vi "Dashboard Main.vi"() -> ()   [LabVIEW 2016]
uses:
  <vilib>/Rock Robotics/WPI/Camera/WPI_CameraExposure Values.ctl
  <vilib>/Rock Robotics/WPI/Camera/WPI_CameraWhite Balance Values.ctl
  <vilib>/Utility/miscctls.llb/LVRowAndColumnTypeDef.ctl
  <vilib>/event_ctls.llb/eventvkey.ctl
  <vilib>/Rock Robotics/Network Tables/NT Read Numeric Array.vi
  <vilib>/Rock Robotics/WPI/Dashboard/WPI_DashboardLogging Global.vi
  <vilib>/Rock Robotics/Network Tables/NT Read Boolean.vi
panel:
  in  "Camera Settings Right":T1={"Frame Rate"=15, "Compression"=30, "Size"=1, "DB Camera Config"=FALSE} {"Frame Rate" scale=1.0..30.0; "Compression" scale=100.0..-1.0; "Size" items=["640x480", "320x240", "160x120"]}
  in  "Camera Name Right":string(combo)="No Camera Selection"
  out "Camera Info":cluster{"Mbps LED":bool, "Mbps":dbl, "fps":dbl} {"fps" format="%#.1g"; "Mbps" format="%#.1g"}
  in  "Camera Settings":T1={"Frame Rate"=10, "Compression"=30, "Size"=1, "DB Camera Config"=FALSE} {"Frame Rate" scale=1.0..30.0; "Compression" scale=100.0..-1.0; "Size" items=["640x480", "320x240", "160x120"]}
  in  "TCP":refnum<k5>
  in  "Rec Mode":enum32{"Stop", "Record", "Playback"}(radio)
  out "Robot IP":string="0.0.0.0"
  out "Image Message":string="Timeout in Camera Communications"
  in  "Dashboard Tab":T2(tab)
  in  "Take Picture":bool
  in  "Vision Target":enum16{"Pegs", "Boiler", "Gears"}(ring)
  in  "Select Auto":string(combo)="Select Autonomous ..."
  out "NT Connection":bool
  out "MotorChart R":cluster{"Numeric":dbl, "Numeric":dbl}(graph)
  out "MotorChart L":cluster{"Numeric":dbl, "Numeric":dbl}(graph)
  out "MotorSliders R":cluster{"MotorSlide1":dbl, "MotorSlide2":dbl} {"MotorSlide2" scale=-1.0..1.0 scale format="%#_2e"; "MotorSlide1" scale=-1.0..1.0 scale format="%#_2e"}
  out "MotorSliders L":cluster{"MotorSlide1":dbl, "MotorSlide2":dbl} {"MotorSlide2" scale=-1.0..1.0 scale format="%#_2e"; "MotorSlide1" scale=-1.0..1.0 scale format="%#_2e"}
  out "Gyro":dbl(knob) scale=0.0..360.0
  out "JS1 Z":dbl(slide) scale=-1.0..1.0 scale format="%#_2e"
  out "JS1 Graph":cluster{"X":dbl, "Y":dbl}[](graph)
  out "JS1 Buttons":T3
  out "JS2 Z":dbl(slide) scale=-1.0..1.0 scale format="%#_2e"
  out "JS2 Graph":cluster{"X":dbl, "Y":dbl}[](graph)
  out "JS2 Buttons":T3
  out "Mode":T4(ring)=enum."Disconnected"
  in  "gear/peg":bool
  out "Binary Image":T5(plugin-control)
  out "Camera Image Right":T5(plugin-control)
  in  "DB/String 9":string
  in  "DB/String 8":string
  in  "DB/String 7":string
  in  "DB/String 6":string
  in  "DB/String 5":string
  in  "DB/String 4":string
  in  "DB/String 3":string
  in  "DB/String 2":string
  in  "DB/String 1":string
  in  "DB/String 0":string
  in  "DB/Slider 0":dbl(slide) scale=0.0..5.0
  in  "DB/Slider 1":dbl(slide) scale=0.0..5.0
  in  "DB/Slider 2":dbl(slide) scale=0.0..5.0
  in  "DB/Slider 3":dbl(slide) scale=0.0..5.0
  out "DB/LED 3":bool
  out "DB/LED 2":bool
  out "DB/LED 1":bool
  out "DB/LED 0":bool
  in  "DB/Button 3":bool
  in  "DB/Button 2":bool
  in  "DB/Button 1":bool
  in  "DB/Button 0":bool caption="New Name"
  in  "Test Slider":dbl(slide) scale=0.0..100.0 scale format="%#_3g"
  in  "On/Off":bool caption="Solenoid"
  in  "Test Name":u16(ring) items=["Select the test to run..."]
  in  "Test Tree":string(tree)
  in  "Motor":cluster{"Value":dbl, "Enable":bool} {"Value" scale=-1.0..1.0 scale format="%#_3g"}
  out "Progress":T6 {"Test Progress" scale=0.0..100.0}
  in  "Rev/Fwd":cluster{"Forward":bool, "Reverse":bool}
  in  "Test Ring":u16(ring) items=["Monochrome", "Color"]
  out "Cmd Status":string
  in  "Execute Command":bool
  in  "Command Params":string[][](table)
  in  "Command Selection":i32(listbox)
  in  "CheckList":i32(listbox)
  out "Tree":string(tree)
  out "Camera Image":T5(plugin-control)
  out "Background":bool
  in  "Camera Name":string(combo)="No Camera Selection"
  # "HW"
  # "HW"
  # "Joysticks"
  # "Drive Motors"
  # "Front"
  # "Right"
  # "Left"
  # "Back"
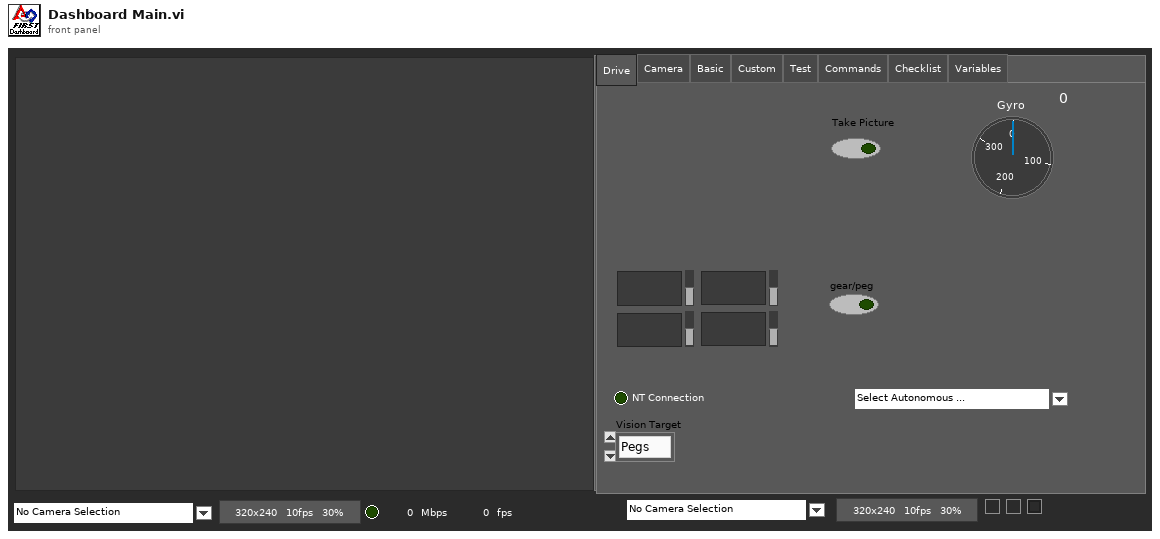
[diagram p1: front panel]
types:
  T1 = cluster{"Frame Rate":i32, "Compression":i32, "Size":u16, "DB Camera Config":bool}
  T2 = enum32{"Drive", "Camera", "Basic", "Custom", "Test", "Commands", "Checklist", "Variables"}
  T3 = cluster{bool, bool, bool, bool, bool, bool, bool, bool, bool, bool, bool, bool}
  T4 = enum8{"Tele-Op Disabled", "Tele-Op Enabled", "Auto Disabled", "Auto Enabled", "Test Disabled", "Test Enabled", "Disconnected", "No Code", "E-Stop"}
  T5 = typedef "IMAQ Image.ctl" = refnum<image>
  T6 = cluster{"Test Progress":u8, "Test Progress Text":string}
  T7 = typedef "Particle Parameters" = i32
  T8 = cluster{"IDs":cluster{"RPC field ID":u16, "Unique ID":u16}, "String":string}
  T9 = enum32{"Drive", "Basic", "Custom", "Test", "Checklist", "Variables"}
  T10 = typedef "Image Type" = u32
  T11 = cluster{"Error Strings":string, "Disable Counts":cluster{u16, u16}, "Rail Faults":cluster{u16, u16, u16}, "Robot IP":string, "DB Mode":u8, "Event Info":cluster{"Name":string, "Type":u8, "Number":u16, "Replay":u8}}
  T12 = cluster{"Storage":cluster{"Disk Free":u64, "RAM Block":u32, "RAM free":u32}, "CPU Utilization":cluster{"CPU % ISR":sgl, "CPU % Time Crit":sgl, "CPU % Timed Str":sgl, "CPU % High":sgl, "CPU % Above":sgl, "CPU % Normal":sgl, "CPU % Low":sgl}, "CAN":cluster{"% Bus Utilization":sgl, "Bus Off Cnt":u32, "TX_FIFO Full Cnt":u32, "Receive Error Cnt":u8, "Transmit Error Cnt":u8}, "HID":cluster{"HID Outputs":u32, "Rumble Low":u16, "Rumble High":u16}[]}
  T13 = cluster{"Status bits":cluster{"Test Mode":bool, "Autonomous":bool, "Enabled":bool, "Code Start":bool, "Brownout":bool, "Reserved 2":bool, "Reserved 3":bool, "E-Stop":bool}, "Code Trace":cluster{"Disabled":bool, "TeleOp":bool, "Auto":bool, "Test":bool}, "Controller Type":enum16{"unknown", "cRIO", "roboRio"}, "Code?":enum16{"unknown", "noCode", "code"}, "Battery V":dbl}
  T14 = cluster{"Control Bits":cluster{"TestMode":bool, "Autonomous":bool, "Enabled":bool, "FMS Present":bool, bool, bool, bool, "E-Stop":bool}, "Team Station ":u8, "Countdown":sgl, "Joystick Values":cluster{"Axes":dbl[], "Buttons":bool[], "POVs":i16[]}[]}
  T15 = cluster{"Axes":dbl[], "Buttons":bool[], "POVs":i16[]}[]
  T16 = cluster{"Axes":dbl[], "Buttons":bool[], "POVs":i16[]}
  T17 = cluster{"Buttons[0]":bool, "Buttons[1]":bool, "Buttons[2]":bool, "Buttons[3]":bool, "Buttons[4]":bool, "Buttons[5]":bool, "Buttons[6]":bool, "Buttons[7]":bool, "Buttons[8]":bool, "Buttons[9]":bool, "Buttons[10]":bool, "Buttons[11]":bool}
  T18 = cluster{"Camera Image":refnum<vi>, "Dashboard Tab":refnum<vi>, "Background":refnum<vi>, "Rec Mode":refnum<vi>, "Test Slider":refnum<vi>, "On/Off ":refnum<vi>, "Test Ring":refnum<vi>, "Rev/Fwd":refnum<vi>, "Test Name":refnum<vi>, "Motor":refnum<vi>, "Progress":refnum<vi>, "CheckList":refnum<vi>, "Tree":refnum<vi>, "Test Tree":refnum<vi>, "Command Params":refnum<vi>, "Command Selection":refnum<vi>, "Execute Command":refnum<vi>, "Cmd Status":refnum<vi>, "Camera Settings":refnum<vi>, "Camera Name":refnum<vi>, "Camera Info":refnum<vi>, "Camera Settings Right":refnum<vi>, "Camera Name Right":refnum<vi>, "Camera Image Right":refnum<vi>}
  T19 = typedef "WPI_CameraExposure Values.ctl" = enum16{"Auto", "Flicker-free 50 Hz", "Flicker-free 60 Hz", "Hold current", "Custom"}
  T20 = typedef "WPI_CameraWhite Balance Values.ctl" = enum16{"Auto", "Fixed indoor", "Fixed outdoor 1", "Fixed outdoor 2", "Fixed fluorescent 1", "Fixed fluorescent 2", "Hold current", "Custom"}
  T21 = cluster{"Exposure":T19, "Exposure (%)":dbl, "Brightness":i32, "White Balance":T20, "Color Temp (K)":dbl}
  T22 = cluster{"Left":dbl, "Top":dbl, "Right":dbl, "Bottom":dbl}
  T23 = cluster{"Numeric":dbl, "Numeric":dbl, "Numeric":dbl, "Numeric":dbl}
  T24 = cluster{"Operation":enum16{"Update", "Clear"}, "Color Box":u32}[]
  T25 = typedef "eventvkey.ctl" = enum16{"ASCII", "Enter", "Return", "Shift", "Ctrl", "Alt", "Cmd", "Opt", "Caps", "NumLock", "Clear", "Break", "Up", "Down", "Left", "Right", "Insert", "Delete", "Home", "End", "PageUp", "PageDown", "Escape", "Help", "Pause", "ScrollLock", "F1", "F2", "F3", "F4", "F5", "F6", "F7", "F8", "F9", "F10", "F11", "F12", "F13", "F14", "F15", "F16", "F17", "F18", "F19", "F20", "F21", "F22", "F23", "F24", "Play", "VolumeUp", "VolumeDown", "Mute", "Two Byte Char"}
  T26 = cluster{"Image Size":bool, "Image Type":bool, "Pixel Value":bool, "ROI Information":bool, "Zoom Factor":bool}
  T27 = cluster{"Operation":enum16{"Update", "Clear"}, "Color Box":u32}
  T28 = typedef "LVRowAndColumnTypeDef.ctl" = cluster{"Row":i32, "Column":i32}
  T29 = cluster{"Shift":bool, "Ctrl":bool, "Alt":bool, "Cmd":bool, "Opt":bool}
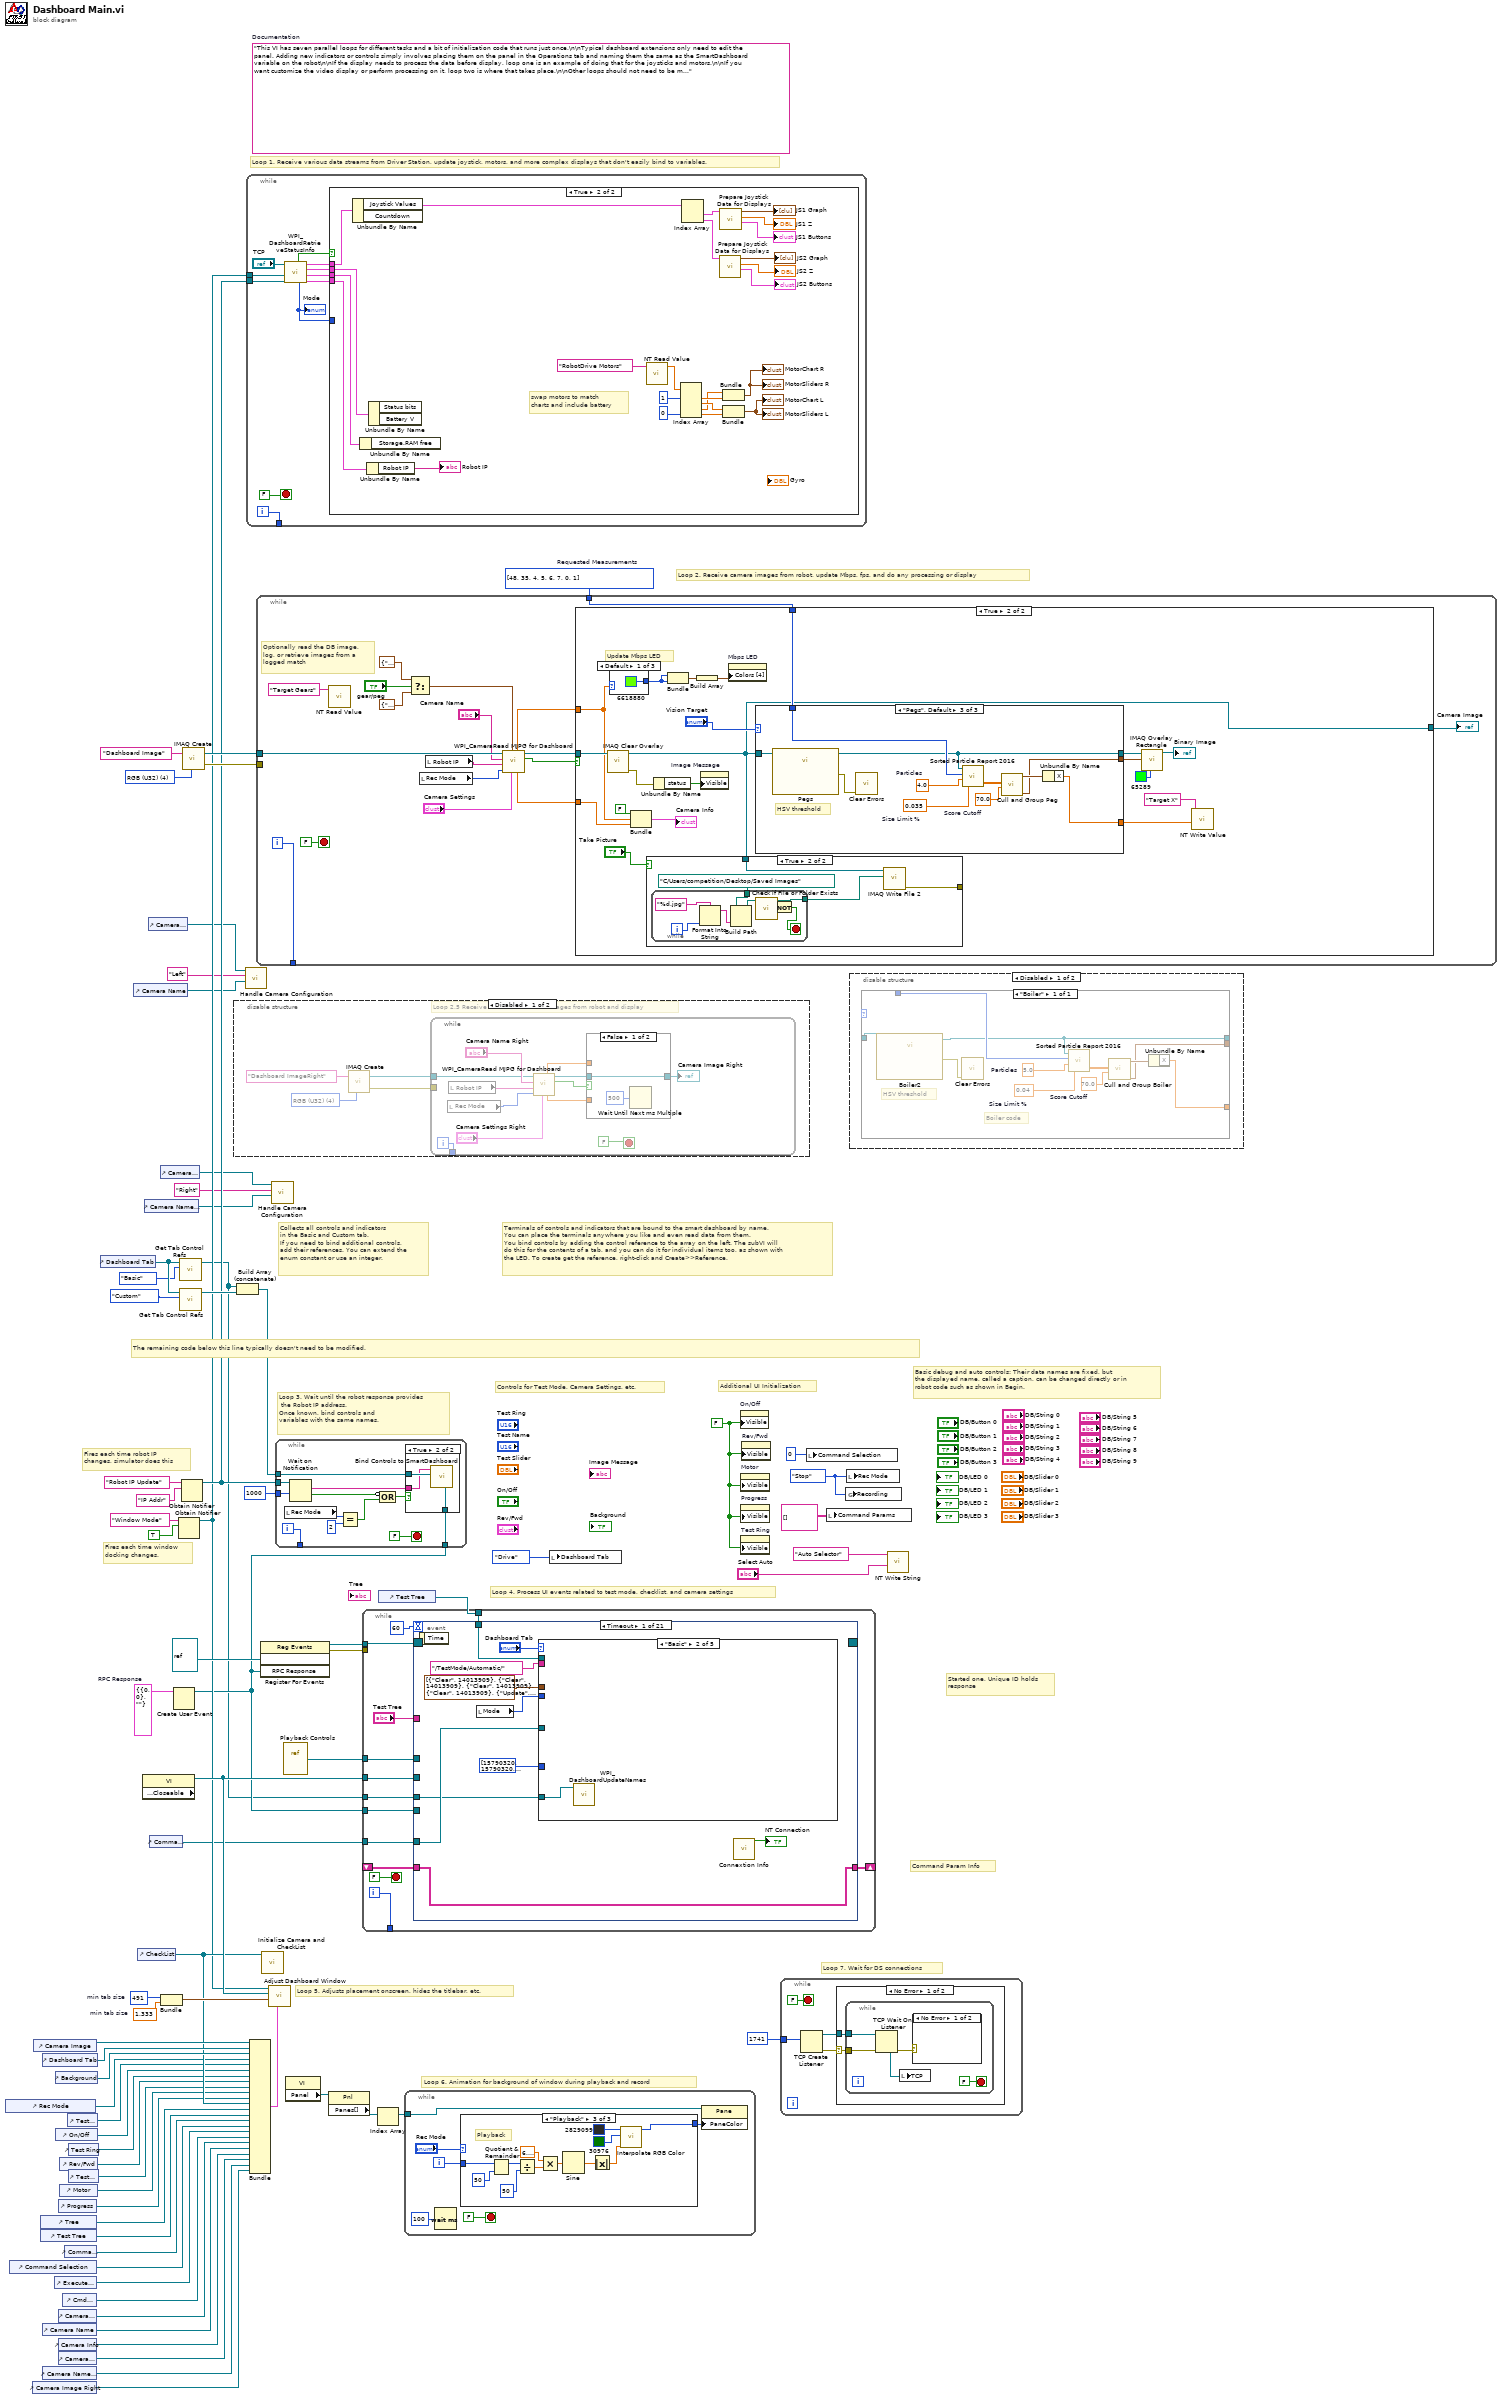
[diagram p0: block diagram]
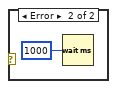
[diagram p5: hidden frame]
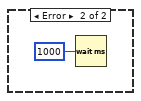
[diagram p6: hidden frame]
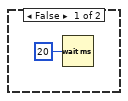
[diagram p7: hidden frame]
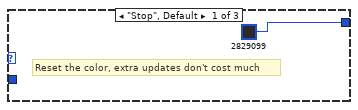
[diagram p8: hidden frame]
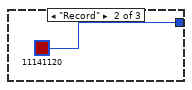
[diagram p9: hidden frame]
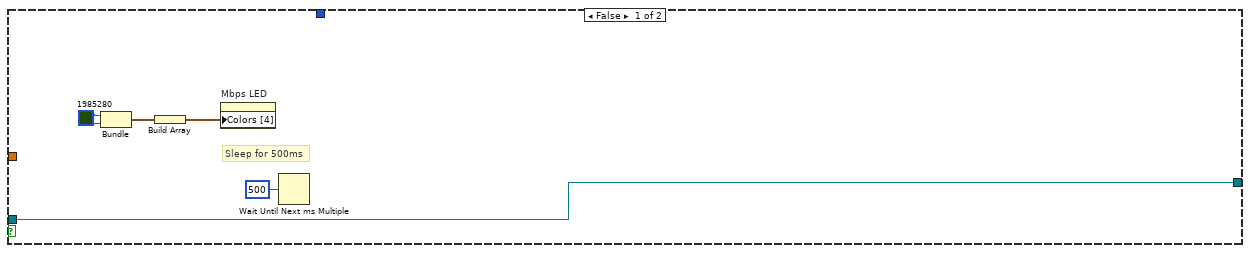
[diagram p11: hidden frame]
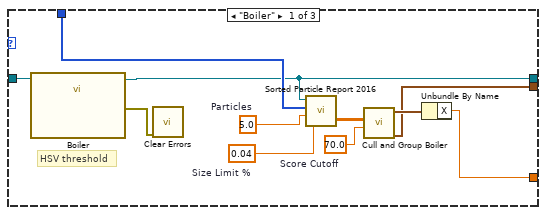
[diagram p13: hidden frame]
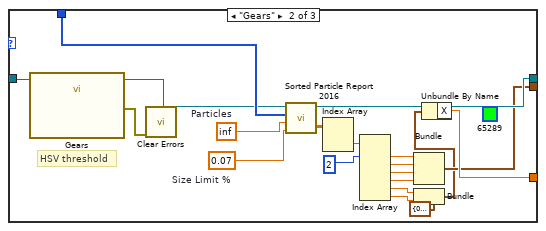
[diagram p14: hidden frame]
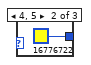
[diagram p15: hidden frame]
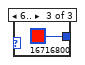
[diagram p16: hidden frame]
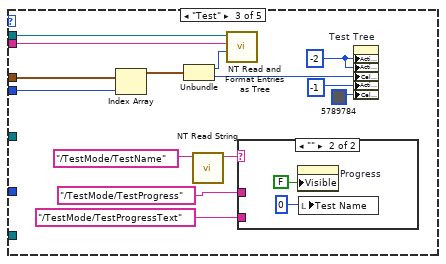
[diagram p18: hidden frame]
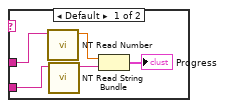
[diagram p19: hidden frame]
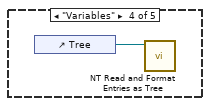
[diagram p20: hidden frame]
diagram:
  w1 = T7[] [48, 35, 4, 5, 6, 7, 0, 1] items=["Center of Mass X", "Center of Mass Y", "First Pixel X", "First Pixel Y", "Bounding Rect Left", "Bounding Rect Top", "Bounding Rect Right", "Bounding Rect Bottom", "Max Feret Diameter Start X", "Max Feret Diameter Start Y", "Max Feret Diameter End X", "Max Feret Diameter End Y", "Max Horiz. Segment Length Left", "Max Horiz. Segment Length Right", "Max Horiz. Segment Length Row", "-", "Bounding Rect Width", "Bounding Rect Height", "Bounding Rect Diagonal", "Perimeter", "Convex Hull Perimeter", "Holes' Perimeter", "Max Feret Diameter", "Equivalent Ellipse Major Axis", "Equivalent Ellipse Minor Axis", "Equivalent Ellipse Minor Axis (Feret)", "Equivalent Rect Long Side", "Equivalent Rect Short Side", "Equivalent Rect Diagonal", "Equivalent Rect Short Side (Feret)", "Average Horiz. Segment Length", "Average Vert. Segment Length", "Hydraulic Radius", "Waddel Disk Diameter", "-", "Area", "Holes' Area", "Particle & Holes' Area", "Convex Hull Area", "Image Area", "-", "Number of Holes", "Number of Horiz. Segments", "Number of Vert. Segments", "-", "Orientation", "Max Feret Diameter Orientation", "-", "% Area/Image Area", "% Area/(Particle & Holes' Area)", "Ratio of Equivalent Ellipse Axes", "Ratio of Equivalent Rect Sides", "-", "Elongation Factor", "Compactness Factor", "Heywood Circularity Factor", "Type Factor", "-", "Sum X", "Sum Y", "Sum XX", "Sum XY", "Sum YY", "Sum XXX", "Sum XXY", "Sum XYY", "Sum YYY", "-", "Moment of Inertia XX", "Moment of Inertia XY", "Moment of Inertia YY", "Moment of Inertia XXX", "Moment of Inertia XXY", "Moment of Inertia XYY", "Moment of Inertia YYY", "Norm. Moment of Inertia XX", "Norm. Moment of Inertia XY", "Norm. Moment of Inertia YY", "Norm. Moment of Inertia XXX", "Norm. Moment of Inertia XXY", "Norm. Moment of Inertia XYY", "Norm. Moment of Inertia YYY", "Hu Moment 1", "Hu Moment 2", "Hu Moment 3", "Hu Moment 4", "Hu Moment 5", "Hu Moment 6", "Hu Moment 7"]  # Requested Measurements
  w23 = T8 {"IDs"={"RPC field ID"=0, "Unique ID"=0}, "String"=""}  # RPC Response
  w48 = 491  # min tab size
  w47 = 1.333  # min tab size
  w55 = enum32{"Stop", "Record", "Playback"}."Stop" ("Rec Mode")
  w30 = FALSE ("Visible")
  (unwired) "This VI has seven parallel loops for different tasks and a bit of initialization code that runs just once.\n\nTypical dashboard extensions only need to edit the panel. Adding new indicators or controls simply involves placing them on the panel in the Operations tab and naming them the same as the SmartDashboard variable on the robot\n\nIf the display needs to process the data before display, loop one is an example of doing that for the joysticks and motors.\n\nIf you want customize the video display or perform processing on it, loop two is where that takes place.\n\nOther loops should not need to be modified. They are pretty standard, and document the task they perform."  # Documentation
  w72 = T10 4 items=["Grayscale (U8)", "Grayscale (I16)", "Grayscale (SGL)", "Complex (CSG)", "RGB (U32)", "HSL (U32)", "RGB (U64)"] ("Image Type")
  # "Command Param Info"
  # "Started one, Unique ID holds\nresponse"
  # "Loop 7. Wait for DS connections"
  # "Basic debug and auto controls: Their data names are fixed, but\nthe displayed name, called a caption, can be changed directly or in\nrobot code such as shown in Begin."
  # "Controls for Test Mode, Camera Settings, etc."
  # "Additional UI Initialization"
  # "Loop 6. Animation for background of window during playback and record"
  # "Fires each time robot IP\nchanges, simulator does this"
  # "Fires each time window\ndocking changes."
  # "Collects all controls and indicators\nin the Basic and Custom tab.\nIf you need to bind additional controls,\nadd their references. You can extend the\nenum constant or use an integer."
  # "The remaining code below this line typically doesn't need to be modified."
  # "Loop 4. Process UI events related to test mode, checklist, and camera settings"
  # "Terminals of controls and indicators that are bound to the smart dashboard by name.\nYou can place the terminals anywhere you like and even read data from them.\nYou bind controls by adding the control reference to the array on the left. The subVI will\ndo this for the contents of a tab, and you can do it for individual items too, as shown with\nthe LED. To create get the reference, right-click and Create>>Reference."
  # "Loop 3. Wait until the robot response provides\n the Robot IP address.\nOnce known, bind controls and\nvariables with the same names."
  # "Loop 5. Adjusts placement onscreen, hides the titlebar, etc."
  # "Loop 1. Receive various data streams from Driver Station, update joystick, motors, and more complex displays that don't easily bind to variables."
  # "Loop 2. Receive camera images from robot, update Mbps, fps, and do any processing or display"
  n1 = control-ref of="Rec Mode"() -> (w36:refnum<vi>)
  n2 = control-ref of="Command Selection"() -> (w22:refnum<vi>)
  n3 = control-ref of="Camera Image Right"() -> (w2:refnum<vi>)
  n4 = control-ref of="Camera Image"() -> (w50:refnum<vi>)
  n5 = control-ref of="Tree"() -> (w40:refnum<vi>)
  n6 = control-ref of="Test Tree"() -> (w39:refnum<vi>)
  n7 = control-ref of="Dashboard Tab"() -> (w49:refnum<vi>)
  n8 = control-ref of="Camera Name"() -> (w13:refnum<vi>)
  n9 = control-ref of="Camera Name Right"() -> (w3:refnum<vi>)
  n10 = control-ref of="Execute Command"() -> (w24:refnum<vi>)
  n11 = control-ref of="Background"() -> (w45:refnum<vi>)
  n12 = control-ref of="On/Off"() -> (w34:refnum<vi>)
  n13 = control-ref of="Progress"() -> (w31:refnum<vi>)
  n14 = control-ref of="Camera Settings"() -> (w14:refnum<vi>)
  n15 = control-ref of="Camera Info"() -> (w12:refnum<vi>)
  n16 = control-ref of="Camera Settings Right"() -> (w4:refnum<vi>)
  n17 = control-ref of="Rev/Fwd"() -> (w32:refnum<vi>)
  n18 = control-ref of="Motor"() -> (w37:refnum<vi>)
  n19 = control-ref of="Cmd Status"() -> (w18:refnum<vi>)
  n20 = control-ref of="Command Params"() -> (w25:refnum<vi>)
  n21 = control-ref of="Test Slider"() -> (w35:refnum<vi>)
  n22 = control-ref of="Test Ring"() -> (w33:refnum<vi>)
  n23 = control-ref of="Test Name"() -> (w38:refnum<vi>)
  n24 = control-ref of="Dashboard Tab"() -> (w53:refnum<vi>)
  n25 = control-ref of="Camera Name"() -> (w15:refnum<vi>)
  n26 = control-ref of="CheckList"() -> (w41:refnum<vi>)
  n27 = property class="VI" props=["Front Panel.Closeable"]() -> (reference out=w54:refnum<vi>)  [unwired: 2 in, 2 out]
  n28 = control-ref of="Camera Name Right"() -> (w7:refnum<vi>)
  n29 = control-ref of="Camera Settings"() -> (w16:refnum<vi>)
  n30 = control-ref of="Command Params"() -> (w17:refnum<vi>)
  n31 = control-ref of="Camera Settings Right"() -> (w8:refnum<vi>)
  n32 = Bundle("min tab size"=w48, "min tab size"=w47) -> (w46:cluster{"min tab size":i32, "min tab size":dbl})  [unwired: 1 in]
  n33 = Create User Event(user event datatype=w23) -> (user event=w19:refnum<user-event>)  [unwired: 1 in, 1 out]
  n34 = Obtain Notifier(name (unnamed)="Window Mode", notification data type=TRUE) -> (notifier out=w28:refnum<notifier>)  [unwired: 2 in, 2 out]
  n35 = call <vilib>:"Get Tab Control Refs.vi"("Page Index"=T9."Basic" ("Dashboard Tab"), "TabControl in"=w53) -> ("ControlsOnPage"=w11:refnum<vi>[])  [unwired: 9 in]
  n36 = call <vilib>:"Get Tab Control Refs.vi"("Page Index"=T9."Custom" ("Dashboard Tab"), "TabControl in"=w53) -> ("ControlsOnPage"=w52:refnum<vi>[])  [unwired: 9 in]
  n37 = Obtain Notifier(name (unnamed)="Robot IP Update", notification data type="IP Addr" ("name (unnamed)")) -> (notifier out=w29:refnum<notifier>)  [unwired: 2 in, 2 out]
  n38 = call "IMAQ Create"("Image Name"="Dashboard Image", "Image Type"=w72) -> ("New Image"=w70:T5, "error out"=w69:errorcluster)  [unwired: 2 in, 1 out]
  n39 = disable-structure shown="Disabled" {
    frame Disabled {
      w75 = T10 4 items=["Grayscale (U8)", "Grayscale (I16)", "Grayscale (SGL)", "Complex (CSG)", "RGB (U32)", "HSL (U32)", "RGB (U64)"] ("Image Type")
      # "Loop 2.5 Receive additional camera images from robot and display"
      n40 = call "IMAQ Create"("Image Name"="Dashboard ImageRight", "Image Type"=w75) -> ("New Image"=w74:T5, "error out"=w73:errorcluster)  [unwired: 2 in, 1 out]
      n41 = while {
        tunnel: w74 -> [w87]
        tunnel: w73 -> [_]
        tunnel: [w81] -> _
        i -> [w81]
        stop <- FALSE stop-if-true
        n42 = local read "Rec Mode"() -> (w85:enum32{"Stop", "Record", "Playback"})
        n43 = local read "Robot IP"() -> (w86:string)
        n44 = call <vilib>:"WPI_CameraRead MJPG for Dashboard.vi"("Camera Settings"="Camera Settings Right", "Rec Mode"=w85, "Robot IP"=w86, "Camera Name"="Camera Name Right", "Refnum in"=w87) -> ("Active"=w80:bool, "Refnum out"=w83:T5, "FPS"=w78:dbl, "Bandwidth (Mbps)"=w79:dbl)  [unwired: 3 in]
        n45 = case shown="False" w80 {
          tunnel: w83 -> [w89 w91]
          tunnel: w79 -> [_ _]
          tunnel: w78 -> [_ _]
          tunnel: [w89 w91] -> w77
          frame False {
            n46 = Wait Until Next ms Multiple(millisecond multiple=u32 500) -> ()  [unwired: 1 out]
          }
          frame True {
          }
        }
        "Camera Image Right" <- w77
      }
    }
    frame Enabled {
    }
  }
  n47 = Build Array (concatenate)(w11, w52) -> (w51:refnum<vi>[])
  n48 = call "Handle Camera Configuration.vi"("CameraNameRef"=w15, "Camera File Name"="Left", "ClusterRef"=w16) -> ()  [unwired: 9 in]
  n49 = while {
    tunnel: [w101] -> _
    tunnel: w29 -> [w95]
    tunnel: w28 -> [w92]
    i -> [w101]
    stop <- FALSE stop-if-true
    n50 = call <vilib>:"WPI_DashboardRetrieveStatusInfo.vi"("Binding Refnum"=w95, "Window Mode Notifier"=w92, "TCP Cnx"="TCP") -> ("Power and Errors"=w96:T11, "Robot Metrics"=w99:T12, "Status Info"=w100:T13, "Control Info"=w97:T14, "Robot Mode"=w94:T4, "Process?"=w98:bool)  [unwired: 3 in]
    "Mode" <- w94
    n51 = case shown="True" w98 {
      tunnel: w100 -> [_ w127]
      tunnel: w99 -> [_ w126]
      tunnel: w97 -> [_ w125]
      tunnel: w96 -> [_ w124]
      tunnel: w94 -> [_ _]
      frame False {
        n52 = Wait (ms)(milliseconds to wait=u32 20) -> ()  [unwired: 1 out]
      }
      frame True {
        # "swap motors to match\ncharts and include battery"
        n53 = Unbundle By Name(w125) -> ("Joystick Values"=w115:T15)  [unwired: 1 out]
        n54 = Unbundle By Name(w126) -> ()  [unwired: 1 out]
        n55 = Unbundle By Name(w124) -> ("Robot IP"=→"Robot IP":string)
        n56 = Unbundle By Name(w127) -> ()  [unwired: 2 out]
        n57 = call-poly <vilib>:"NT Read Value.vi"("Name"="RobotDrive Motors") -> ("Numeric Array"=w105:dbl[])  [unwired: 9 in, 1 out]
        n58 = Index Array(array=w105, index #1=1, index #4=0) -> (element #1=w119:dbl, element #2=w120:dbl, element #3=w118:dbl, element #4=w123:dbl)  [unwired: 2 in]
        n59 = Index Array(array=w115) -> (element #1=w114:T16, element #2=w110:T16)  [unwired: 2 in]
        n60 = call "Prepare Joystick Data for Displays.vi"("Joystick Values"=w110) -> ("Buttons"=→"JS2 Buttons":T17, "Z Axis"=→"JS2 Z":dbl, "Cartesian Data"=→"JS2 Graph":cluster{"X axis":dbl, "X axis":dbl}[])  [unwired: 8 in]
        n61 = call "Prepare Joystick Data for Displays.vi"("Joystick Values"=w114) -> ("Buttons"=→"JS1 Buttons":T17, "Z Axis"=→"JS1 Z":dbl, "Cartesian Data"=→"JS1 Graph":cluster{"X axis":dbl, "X axis":dbl}[])  [unwired: 8 in]
        n62 = Bundle("Numeric"=w118, "Numeric"=w119) -> (→"MotorChart R" →"MotorSliders R":cluster{"Numeric":dbl, "Numeric":dbl})  [unwired: 1 in]
        n63 = Bundle("Numeric"=w120, "Numeric"=w123) -> (→"MotorChart L" →"MotorSliders L":cluster{"Numeric":dbl, "Numeric":dbl})  [unwired: 1 in]
      }
    }
  }
  n64 = Bundle("Camera Image"=w50, "Dashboard Tab"=w49, "Background"=w45, "Rec Mode"=w36, "Test Slider"=w35, "On/Off"=w34, "Test Ring"=w33, "Rev/Fwd"=w32, "Test Name"=w38, "Motor"=w37, "Progress"=w31, "CheckList"=w41, "Tree"=w40, "Test Tree"=w39, "Command Params"=w25, "Command Selection"=w22, "Execute Command"=w24, "Cmd Status"=w18, "Camera Settings"=w14, "Camera Name"=w13, "Camera Info"=w12, "Camera Settings Right"=w4, "Camera Name Right"=w3, "Camera Image Right"=w2) -> (w42:T18)  [unwired: 1 in]
  n65 = while {
    tunnel: w70 -> [w143]
    tunnel: w69 -> [_]
    tunnel: [w144] -> _
    tunnel: w1 -> [w134]
    i -> [w144]
    stop <- FALSE stop-if-true
    # "Optionally read the DB image,\nlog, or retrieve images from a\nlogged match"
    n66 = call-poly <vilib>:"NT Read Value.vi"("Name"="Target Gears") -> ()  [unwired: 9 in, 2 out]
    n67 = Select(t=T21 {"Exposure"=enum."Custom", "Exposure (%)"=35.0, "Brightness"=50, "White Balance"=enum."Custom", "Color Temp (K)"=0.0} ("Bright"), s="gear/peg", f=T21 {"Exposure"=enum."Custom", "Exposure (%)"=0.0, "Brightness"=0, "White Balance"=enum."Custom", "Color Temp (K)"=0.0} ("Dark")) -> (s? t:f=w132:T21)
    n68 = local read "Rec Mode"() -> (w140:enum32{"Stop", "Record", "Playback"})
    n69 = local read "Robot IP"() -> (w139:string)
    n70 = call <vilib>:"WPI_CameraRead MJPG for Dashboard.vi"("Camera Settings"="Camera Settings", "Camera Settings 2"=w132, "Rec Mode"=w140, "Robot IP"=w139, "Camera Name"="Camera Name", "Refnum in"=w143) -> ("Active"=w142:bool, "Refnum out"=w129:T5, "FPS"=w141:dbl, "Bandwidth (Mbps)"=w138:dbl)  [unwired: 2 in]
    n71 = case shown="True" w142 {
      tunnel: w129 -> [w146 w166]
      tunnel: w138 -> [_ w163]
      tunnel: w141 -> [_ w164]
      tunnel: [w146 w153] -> w135
      tunnel: w134 -> [_ w160]
      frame False {
        w148 = u32 1985280 ("Color Box")
        # "Sleep for 500ms"
        n72 = Bundle("Color Box"=w148, "Color Box"=w148) -> (w149:cluster{"Color Box":u32, "Color Box":u32})  [unwired: 1 out]
        n73 = Build Array(w149) -> (w147:cluster{"Color Box":u32, "Color Box":u32}[])
        n74 = property on="Mbps LED" class="Bool (strict)"("Colors [4]"=w147) -> ()  [unwired: 2 in, 2 out]
        n75 = Wait Until Next ms Multiple(millisecond multiple=u32 500) -> ()  [unwired: 1 out]
      }
      frame True {
        # "Update Mbps LED"
        n76 = call "IMAQ Clear Overlay"("Image"=w166) -> ("error out"=w169:errorcluster, "Image Out"=w153:T5)  [unwired: 2 in, 7 out]
        n77 = case shown="Default" w163 {
          tunnel: [u32 6618880 ("Color Box") u32 16776722 ("Color Box") u32 16716800 ("Color Box")] -> w167
          frame Default {
          }
          frame 4, 5 {
          }
          frame 6.. {
          }
        }
        n78 = Bundle(FALSE, "Bandwidth (Mbps)"=w163, "FPS"=w164) -> (→"Camera Info":cluster{bool, "Bandwidth (Mbps)":dbl, "FPS":dbl})  [unwired: 1 in]
        n79 = case shown="True" "Take Picture" {
          tunnel: w153 -> [_ w174]
          tunnel: [_ w173] -> _
          frame False {
          }
          frame True {
            n80 = while {
              tunnel: path "C:/Users/competition/Desktop/Saved Images" ("base path") -> [w179]
              tunnel: [w177] -> w171
              i -> [w181]
              stop <- w176 stop-if-true
              n81 = Format Into String(format string="%d.jpg", w181) -> (resulting string=w180:string)  [unwired: 2 in, 1 out]
              n82 = Build Path(base path=w179, name or relative path=w180) -> (appended path=w178:path)
              n83 = call <vilib>:"Check if File or Folder Exists.vi"("path"=w178) -> ("file or folder exists?"=w182:bool, "dup path"=w177:path)  [unwired: 8 in, 1 out]
              n84 = Not(x=w182) -> (.not. x?=w176:bool)
            }
            n85 = call-poly "IMAQ Write File 2"("File Path"=w171, "Image"=w174) -> ("error out"=w173:errorcluster)  [unwired: 3 in, 6 out]
          }
        }
        n86 = Unbundle By Name(w169) -> ("status"=w170:bool)
        n87 = Bundle("Color Box"=w167, "Color Box"=w167) -> (w168:cluster{"Color Box":u32, "Color Box":u32})  [unwired: 1 out]
        n88 = Build Array(w168) -> (w165:cluster{"Color Box":u32, "Color Box":u32}[])
        n89 = property on="Image Message" class="Str"("Visible"=w170) -> ()  [unwired: 2 in, 2 out]
        n90 = property on="Mbps LED" class="Bool (strict)"("Colors [4]"=w165) -> ()  [unwired: 2 in, 2 out]
        n91 = case shown="\"Pegs\", Default" "Vision Target" {
          tunnel: w160 -> [w190 w207 w221]
          tunnel: [w186 w212 w220] -> w151
          tunnel: w153 -> [w185 w210 w219]
          tunnel: [w183 w206 w214] -> w156
          tunnel: [w184 w198 w215] -> w154
          frame "Boiler" {
            w188 = 70.0  # Score Cutoff
            w192 = 5.0  # Particles
            w191 = 0.04  # Size Limit %
            # "HSV threshold"
            n92 = call "Boiler"("Image In"=w185) -> ("Image Out"=w183:T5, "error out"=w193:errorcluster)  [unwired: 25 in]
            n93 = call <vilib>:"Clear Errors.vi"("error in (no error)"=w193) -> ()  [unwired: 5 in, 2 out]
            n94 = call "Sorted Particle Report 2016.vi"("Min Area Size %"=w191, "Particle Count Limit"=w192, "Pixel Measurements"=w190, "Image in"=w183) -> ("Sorted Data"=w189:dbl[][])  [unwired: 1 out]
            n95 = call "Cull and Group Boiler.vi"("Score Cutoff"=w188, "Sorted Data"=w189) -> ("Rect"=w184:T22, "Center"=w187:cluster{"X":dbl, "Y":dbl})  [unwired: 6 in, 2 out]
            n96 = Unbundle By Name(w187) -> ("X"=w186:dbl)
          }
          frame "Gears" {
            w209 = inf  # Particles
            w208 = 0.07  # Size Limit %
            (unwired) u32 65289 ("Color")
            # "HSV threshold"
            n97 = call "Gears"("Image In"=w210) -> ("Image Out"=w206:T5, "error out"=w211:errorcluster)  [unwired: 25 in]
            n98 = call <vilib>:"Clear Errors.vi"("error in (no error)"=w211) -> ()  [unwired: 5 in, 2 out]
            n99 = call "Sorted Particle Report 2016.vi"("Min Area Size %"=w208, "Particle Count Limit"=w209, "Pixel Measurements"=w207, "Image in"=w206) -> ("Sorted Data"=w205:dbl[][])  [unwired: 1 out]
            n100 = Index Array(array=w205) -> (element=w204:dbl[])  [unwired: 2 in]
            n101 = Index Array(array=w204, index #1=2 ("index")) -> (element #1=w202:dbl, element #2=w201:dbl, element #3=w200:dbl, element #4=w199:dbl, element #5=w196:dbl, element #6=w197:dbl)  [unwired: 5 in]
            n102 = Bundle("Numeric"=w202, "Numeric"=w201, "Numeric"=w200, "Numeric"=w199) -> (w198:T23)  [unwired: 1 in]
            n103 = Bundle(cluster=cluster{"X":dbl, "Y":dbl} {"X"=0.0, "Y"=0.0} ("input cluster"), "X"=w196, "Y"=w197) -> (w194:cluster{"X":dbl, "Y":dbl})
            n104 = Unbundle By Name(w194) -> ("X"=w212:dbl)
          }
          frame "Pegs", Default {
            w216 = 70.0  # Score Cutoff
            w223 = 4.0  # Particles
            w222 = 0.035  # Size Limit %
            # "HSV threshold"
            n105 = call "Pegs"("Image In"=w219) -> ("Image Out"=w214:T5, "error out"=w213:errorcluster)  [unwired: 25 in]
            n106 = call <vilib>:"Clear Errors.vi"("error in (no error)"=w213) -> ()  [unwired: 5 in, 2 out]
            n107 = call "Sorted Particle Report 2016.vi"("Min Area Size %"=w222, "Particle Count Limit"=w223, "Pixel Measurements"=w221, "Image in"=w214) -> ("Sorted Data"=w218:dbl[][])  [unwired: 1 out]
            n108 = call "Cull and Group Peg.vi"("Score Cutoff"=w216, "Sorted Data"=w218) -> ("Rect"=w215:T22, "Center"=w217:cluster{"X":dbl, "Y":dbl})  [unwired: 6 in, 2 out]
            n109 = Unbundle By Name(w217) -> ("X"=w220:dbl)
          }
        }
        n110 = call "IMAQ Overlay Rectangle"("Color"=u32 65289, "Rectangle"=w154, "Image"=w156) -> ("Image Out"=→"Binary Image":T5)  [unwired: 7 in, 1 out]
        n111 = call-poly <vilib>:"NT Write Value.vi"("Numeric"=w151, "Name"="Target X") -> ()  [unwired: 9 in, 1 out]
      }
    }
    "Camera Image" <- w135
  }
  n112 = register-events(refnum<vi> refnum, w19) -> (reference out=w59:refnum<event-registration>, error out=w58:errorcluster)  [unwired: 2 in]
  n113 = call "Initialize Camera and CheckList.vi"("ListBox in"=w41) -> ()  [unwired: 11 in]
  n114 = call "Adjust Dashboard Window.vi"("Sizing Refnums"=w42, "Size Constraints"=w46, "VI"=w54, "WIn Mode"=w28) -> ()  [unwired: 8 in]
  n115 = call "Handle Camera Configuration.vi"("CameraNameRef"=w7, "Camera File Name"="Right", "ClusterRef"=w8) -> ()  [unwired: 9 in]
  n116 = while {
    tunnel: w51 -> [w238]
    tunnel: w29 -> [w236]
    tunnel: [w234] -> _
    tunnel: u32 1000 ("milliseconds to wait") -> [w233]
    tunnel: w19 -> [w227]
    i -> [w234]
    stop <- FALSE stop-if-true
    n117 = local read "Rec Mode"() -> (w229:enum32{"Stop", "Record", "Playback"})
    n118 = Wait on Notification(notifier=w236, timeout in ms (-1)=w233) -> (notification=w235:string, timed out?=w231:bool)  [unwired: 2 in, 2 out]
    n119 = Equal?(x=w229, y=u16 2 ("Rec Mode")) -> (x = y?=w230:bool)
    n120 = Compound Arithmetic op=OR(invert w231, w230) -> (w232:bool)
    n121 = case shown="True" w232 {
      tunnel: w238 -> [_ w241]
      tunnel: w235 -> [_ w240]
      tunnel: w227 -> [_ w239]
      frame False {
      }
      frame True {
        n122 = call <vilib>:"Bind Controls to SmartDashboard.vi"("RPC ref"=w239, "Bound Control Refs"=w241, "Server IP Address"=w240) -> ()  [unwired: 9 in]
      }
    }
  }
  n123 = vi-ref "Playback Controls.vi"() -> (w60:refnum<vi>)
  n124 = property class="VI"() -> ("Panel"=w62:refnum<vi>)  [unwired: 2 in, 2 out]
  n125 = property class="Pnl"(reference=w62) -> ("Panes[]"=w63:refnum<vi>[])  [unwired: 1 in, 2 out]
  n126 = Index Array(array=w63) -> (element=w61:refnum<vi>)  [unwired: 1 in]
  n127 = control-ref of="Test Tree"() -> (w64:refnum<vi>)
  n128 = while {
    tunnel: [w251] -> _
    tunnel: w64 -> [w250]
    tunnel: w60 -> [w249]
    tunnel: w59 -> [w248]
    tunnel: w58 -> [_]
    tunnel: w54 -> [w247]
    tunnel: w19 -> [w246]
    tunnel: w17 -> [w245]
    shift-right: [w244] -> _
    shift-left: _ -> [w243]
    tunnel: w11 -> [w242]
    i -> [w251]
    stop <- FALSE stop-if-true
    n129 = event shown="[0] Timeout" {
      selector: w248 -> [_ _ _ _ _ _ _ _ _ _ _ _ _ _ _ _ _ _ _ _ _]
      dyn-events: [_ _ _ _ _ _ _ _ _ _ _ _ _ _ _ _ w507 _ _ _ _] -> _
      timeout: u32 60 ("milliseconds to wait") -> [_ _ _ _ _ _ _ _ _ _ _ _ _ _ _ _ _ _ _ _ _]
      tunnel: w250 -> [w263 _ _ _ _ _ _ _ _ _ _ _ _ _ _ _ _ _ _ _ _]
      tunnel: "Test Tree" -> [_ _ _ _ _ _ _ _ _ _ _ w474 w482 w484 w488 w496 _ _ _ _ _]
      tunnel: w249 -> [_ _ _ _ _ _ _ _ _ _ _ _ _ _ _ _ w509 _ w527 _ _]
      tunnel: w247 -> [_ _ _ _ _ _ _ _ _ _ _ _ _ _ _ _ w505 _ _ _ _]
      tunnel: w246 -> [_ _ _ _ _ _ _ _ _ _ _ _ _ _ _ _ w501 _ _ _ _]
      tunnel: w245 -> [w258 _ _ _ _ _ w425 _ _ _ _ _ _ _ _ _ _ _ _ _ _]
      tunnel: [w257 w302 w404 w409 w418 w422 w423 w432 w442 w449 w461 w473 w480 w483 w487 w495 w500 w522 w524 w528 w539] -> w244
      tunnel: w243 -> [w257 w302 w404 w409 w418 w422 w423 _ _ w449 w461 w473 w480 w483 w487 w495 w500 w522 w524 w528 w539]
      tunnel: w242 -> [w255 _ _ _ _ _ _ _ _ _ _ _ _ _ _ _ _ _ _ _ _]
      event Timeout {
        n130 = event-data() -> ()  [unwired: 1 in, 1 out]
        n131 = local read "Mode"() -> (w260:T4)
        n132 = case shown="\"Basic\"" "Dashboard Tab" {
          tunnel: w263 -> [_ _ w279 _ _]
          tunnel: "/TestMode/Automatic/" ("Name Pattern") -> [_ _ w278 _ _]
          tunnel: T24 [{"Operation"=enum."Clear", "Color Box"=14013909}, {"Operation"=enum."Clear", "Color Box"=14013909}, {"Operation"=enum."Clear", "Color Box"=14013909}, {"Operation"=enum."Clear", "Color Box"=14013909}, {"Operation"=enum."Update", "Color Box"=14013909}, {"Operation"=enum."Update", "Color Box"=16777215}, {"Operation"=enum."Clear", "Color Box"=14013909}, {"Operation"=enum."Clear", "Color Box"=14013909}, {"Operation"=enum."Clear", "Color Box"=14013909}] -> [_ _ w271 _ w295]
          tunnel: w260 -> [_ _ w270 _ w294]
          tunnel: u32[] [15790320, 15790320, 15790320, 15790320, 16777215, 16777215, 15790320, 15790320, 15790320] -> [_ _ _ _ w300]
          tunnel: w258 -> [_ _ _ _ w288]
          tunnel: w255 -> [_ w265 _ _ _]
          frame "Custom", Default {
          }
          frame "Basic" {
            n133 = call <vilib>:"WPI_DashboardUpdateNames.vi"("Controls on Tab"=w265) -> ()  [unwired: 11 in]
          }
          frame "Test" {
            w277 = -2 ("Active Item:Row Number")
            n134 = Index Array(array=w271, index=w270) -> (element=w272:T27)
            n135 = Unbundle(w272) -> ("Operation"=w273:enum16{"Update", "Clear"}, "Color Box"=w274:u32)
            n136 = call <vilib>:"NT Read String.vi"("Name"="/TestMode/TestName") -> ("String"=w268:string)  [unwired: 9 in, 1 out]
            n137 = call <vilib>:"NT Read and Format Entries as Tree.vi"("Operation"=w273, "Name Pattern"=w278, "Tree Refnum"=w279) -> ()  [unwired: 7 in, 2 out]
            n138 = case shown="\"\"" w268 {
              tunnel: "/TestMode/TestProgress" ("Name") -> [w281 _]
              tunnel: "/TestMode/TestProgressText" ("Name") -> [w280 _]
              frame Default {
                n139 = call <vilib>:"NT Read Number.vi"("Name"=w281) -> ("Numeric"=w282:dbl)  [unwired: 9 in, 1 out]
                n140 = call <vilib>:"NT Read String.vi"("Name"=w280) -> ("String"=w283:string)  [unwired: 9 in, 1 out]
                n141 = Bundle("Numeric"=w282, "String"=w283) -> (→"Progress":cluster{"Numeric":dbl, "String":string})  [unwired: 1 in]
              }
              frame "" {
                n142 = property on="Progress" class="Clust (strict)"("Visible"=FALSE) -> ()  [unwired: 2 in, 2 out]
                n143 = local write "Test Name"(u16 0) -> ()
              }
            }
            n144 = property on="Test Tree" class="Tree (strict)"("Active Item Row Number"=w277, "ActiveColNum"=w277, "CellBG"=w274, "Active Item Row Number"=-1 ("Active Item:Row Number"), "CellBG"=u32 5789784 ("Color Box")) -> ()  [unwired: 2 in, 2 out]
          }
          frame "Variables" {
            n145 = control-ref of="Tree"() -> (w287:refnum<vi>)
            n146 = call <vilib>:"NT Read and Format Entries as Tree.vi"("Tree Refnum"=w287) -> ()  [unwired: 9 in, 2 out]
          }
          frame "Commands" {
            w296 = u32 5789784 ("Color Box")
            w297 = T28 {"Row"=-1, "Column"=-2} ("Active Cell:Active Cell")
            w299 = T28 {"Row"=-2, "Column"=-2} ("Active Cell:Active Cell")
            n147 = Index Array(array=w300, index=w294) -> (element=w298:u32)
            n148 = Index Array(array=w295, index=w294) -> (element=w293:T27)
            n149 = Unbundle(w293) -> ("Operation"=w292:enum16{"Update", "Clear"})  [unwired: 1 out]
            n150 = local read "Command Selection"() -> (w291:i32)
            n151 = property on="Command Selection" class="MCListbox (strict)"("ActiveCell"=w299, "CellBG"=w298, "ActiveCell"=w297, "CellBG"=w296) -> ()  [unwired: 2 in, 2 out]
            n152 = call <vilib>:"WPI_DashboardUpdate RPC Info.vi"("Operation"=w292) -> ("update"=w290:bool, "commands"=w289:string[][])  [unwired: 9 in]
            n153 = property on="Command Selection" class="MCListbox (strict)"("ItemNames"=w289) -> ()  [unwired: 2 in, 2 out]
            n154 = property on="Command Params" class="Tbl (strict)"("Active Cell"=w299, "Cell BG Color"=w298, "Active Cell"=w297, "Cell BG Color"=w296) -> ()  [unwired: 2 in, 2 out]
            n155 = call <vilib>:"WPI_DashboardUpdate Command Params.vi"("Update"=w290, "NewVal"=w291, "Commands"=w289, "Param Tbl"=w288) -> ()  [unwired: 7 in, 1 out]
          }
        }
        n156 = call <vilib>:"Connextion Info.vi"() -> ("Connected"=→"NT Connection":bool)  [unwired: 10 in, 1 out]
      }
      event "Test Tree": Value Change {
        # "Show appropriate\ncontrols"
        n157 = event-data() -> ("CtlRef"=w305:refnum<vi>, "NewVal"=w303:string)  [unwired: 1 in]
        n158 = call <vilib>:"WPI_UtilitiesGetTreeIOName.vi"("NewVal"=w303, "TreeControl in"=w305) -> ("I/O Name"=w306:string)  [unwired: 9 in]
        n159 = case shown="\"Camera\"" w306 {
          selector: w306 -> [_ w313 _ w335 w344 _]
          tunnel: w303 -> [_ _ w332 w334 _ w351]
          tunnel: cluster{string[]}[] [{["640x480", "320x240", "160x120"]}, {["Auto", "Fixed indoor", "Fixed outdoor 1", "Fixed outdoor 2", "Fixed fluorescent 1", "Fixed fluorescent 2", "Hold current"]}, {["Auto", "Flicker-free 50 Hz", "Flicker-free 60 Hz", "Hold current"]}, {["None", "Prioritize frame rate", "Prioritize image quality"]}, {["Monochrome", "Color"]}] -> [_ _ _ _ _ w350]
          frame Default {
            w308 = FALSE ("Visible")
            w307 = FALSE ("Visible")
            n160 = property on="Motor" class="Clust (strict)"("Visible"=w307) -> ()  [unwired: 2 in, 2 out]
            n161 = property on="Test Ring" class="Ring (strict)"("Visible"=w307) -> ()  [unwired: 2 in, 2 out]
            n162 = property on="Rev/Fwd" class="Clust (strict)"("Visible"=w308) -> ()  [unwired: 2 in, 2 out]
            n163 = property on="On/Off" class="Bool (strict)"("Visible"=w308) -> ()  [unwired: 2 in, 2 out]
            n164 = property on="Test Slider" class="Slide (strict)"("Visible"=w308) -> ()  [unwired: 2 in, 2 out]
          }
          frame "Analog Out", "Motor", "PWM" {
            w314 = FALSE ("Visible")
            n165 = case shown="\"Analog Out\"" w313 {
              tunnel: [1.0 ("Value") -1.0 ("Value") 0.0 ("Value")] -> w312
              tunnel: [255.0 ("Value") 1.0 ("Value") 5.0 ("Value")] -> w311
              tunnel: [128.0 ("Value") 0.0 ("Value") 0.0 ("Value")] -> w310
              tunnel: [64.0 ("Value") 0.5 ("Value") 1.0 ("Value")] -> w309
              frame "PWM" {
              }
              frame "Motor", Default {
              }
              frame "Analog Out" {
              }
            }
            n166 = property on="Motor" class="Clust (strict)"("Visible"=TRUE) -> ()  [unwired: 2 in, 2 out]
            n167 = property on="Value" class="Slide (strict)"("Value"=w310, "Scale.Minimum"=w312, "Scale.Maximum"=w311, "Scale.Increment"=w309) -> ()  [unwired: 2 in, 2 out]
            n168 = property on="On/Off" class="Bool (strict)"("Visible"=w314) -> ()  [unwired: 2 in, 2 out]
            n169 = property on="Test Slider" class="Slide (strict)"("Visible"=w314) -> ()  [unwired: 2 in, 2 out]
            n170 = property on="Test Ring" class="Ring (strict)"("Visible"=w314) -> ()  [unwired: 2 in, 2 out]
            n171 = property on="Rev/Fwd" class="Clust (strict)"("Visible"=w314) -> ()  [unwired: 2 in, 2 out]
          }
          frame "Servo" {
            w330 = FALSE ("Visible")
            n172 = call <vilib>:"NT Read Number.vi"("Name"=w332) -> ("Numeric"=w331:dbl)  [unwired: 9 in, 1 out]
            n173 = property on="Test Slider" class="Slide (strict)"("Visible"=TRUE, "Scale.Maximum"=170.0 ("Scale.Range:Maximum")) -> ()  [unwired: 2 in, 2 out]
            n174 = local write "Test Slider"(w331) -> ()
            n175 = property on="Motor" class="Clust (strict)"("Visible"=w330) -> ()  [unwired: 2 in, 2 out]
            n176 = property on="Rev/Fwd" class="Clust (strict)"("Visible"=w330) -> ()  [unwired: 2 in, 2 out]
            n177 = property on="On/Off" class="Bool (strict)"("Visible"=w330) -> ()  [unwired: 2 in, 2 out]
            n178 = property on="Test Ring" class="Ring (strict)"("Visible"=w330) -> ()  [unwired: 2 in, 2 out]
          }
          frame "Relay", "Solenoid" {
            w333 = FALSE ("Visible")
            n179 = property on="Motor" class="Clust (strict)"("Visible"=w333) -> ()  [unwired: 2 in, 2 out]
            n180 = property on="Test Slider" class="Slide (strict)"("Visible"=w333) -> ()  [unwired: 2 in, 2 out]
            n181 = Search and Replace String(input string=w334, search string="/Value  **", replace string="/Direction") -> (result string=w340:string)  [unwired: 5 in, 3 out]
            n182 = property on="Test Ring" class="Ring (strict)"("Visible"=w333) -> ()  [unwired: 2 in, 2 out]
            n183 = call <vilib>:"NT Read String.vi"("Name"=w340) -> ("String"=w338:string)  [unwired: 9 in, 1 out]
            n184 = Equal?(x="Both directions", y=w338) -> (x = y?=w336:bool)
            n185 = Not(x=w336) -> (.not. x?=w337:bool)
            n186 = property on="Rev/Fwd" class="Clust (strict)"("Visible"=w336) -> ()  [unwired: 2 in, 2 out]
            n187 = property on="On/Off" class="Bool (strict)"("Visible"=w337, "Caption.Text"=w335) -> ()  [unwired: 2 in, 2 out]
          }
          frame "Compressor", "Digital Out" {
            w343 = FALSE ("Visible")
            # "Get direction and finish"
            n188 = property on="Motor" class="Clust (strict)"("Visible"=w343) -> ()  [unwired: 2 in, 2 out]
            n189 = property on="Test Slider" class="Slide (strict)"("Visible"=w343) -> ()  [unwired: 2 in, 2 out]
            n190 = property on="Test Ring" class="Ring (strict)"("Visible"=w343) -> ()  [unwired: 2 in, 2 out]
            n191 = property on="On/Off" class="Bool (strict)"("Visible"=TRUE, "Caption.Text"=w344) -> ()  [unwired: 2 in, 2 out]
            n192 = property on="Rev/Fwd" class="Clust (strict)"("Visible"=FALSE) -> ()  [unwired: 2 in, 2 out]
          }
          frame "Camera" {
            n193 = call <vilib>:"Get Last Path Segment.vi"("String in"=w351) -> ("String out"=w352:string)  [unwired: 10 in]
            n194 = property on="On/Off" class="Bool (strict)"("Visible"=FALSE) -> ()  [unwired: 2 in, 2 out]
            n195 = property on="Motor" class="Clust (strict)"("Visible"=FALSE) -> ()  [unwired: 2 in, 2 out]
            n196 = property on="Rev/Fwd" class="Clust (strict)"("Visible"=FALSE) -> ()  [unwired: 2 in, 2 out]
            n197 = case shown="\"White Balance  **\"" w352 {
              tunnel: w351 -> [w358 w367 w376 w385 w394 _ w400]
              tunnel: w350 -> [w356 w364 w373 w382 w391 _ _]
              frame "Size  **" {
                n198 = Index Array(array=w356) -> (element=w355:cluster{string[]})  [unwired: 1 in]
                n199 = call <vilib>:"NT Read String.vi"("Name"=w358) -> ("String"=w357:string)  [unwired: 9 in, 1 out]
                n200 = Unbundle(w355) -> (w353:string[])
                n201 = Match First String(2:w353, 3:w357) -> (0:w354:i32)  [unwired: 1 out]
                n202 = property on="Test Ring" class="Ring (strict)"("Value"=w354, "Strings []"=w353) -> ()  [unwired: 2 in, 2 out]
                n203 = property on="Test Ring" class="Ring (strict)"("Visible"=TRUE) -> ()  [unwired: 2 in, 2 out]
                n204 = property on="Test Slider" class="Slide (strict)"("Visible"=FALSE) -> ()  [unwired: 2 in, 2 out]
              }
              frame "White Balance  **" {
                n205 = Index Array(array=w364, index=1) -> (element=w365:cluster{string[]})
                n206 = call <vilib>:"NT Read String.vi"("Name"=w367) -> ("String"=w366:string)  [unwired: 9 in, 1 out]
                n207 = Unbundle(w365) -> (w362:string[])
                n208 = Match First String(2:w362, 3:w366) -> (0:w361:i32)  [unwired: 1 out]
                n209 = property on="Test Ring" class="Ring (strict)"("Value"=w361, "Strings []"=w362) -> ()  [unwired: 2 in, 2 out]
                n210 = property on="Test Ring" class="Ring (strict)"("Visible"=TRUE) -> ()  [unwired: 2 in, 2 out]
                n211 = property on="Test Slider" class="Slide (strict)"("Visible"=FALSE) -> ()  [unwired: 2 in, 2 out]
              }
              frame "Exposure  **" {
                n212 = Index Array(array=w373, index=2) -> (element=w374:cluster{string[]})
                n213 = call <vilib>:"NT Read String.vi"("Name"=w376) -> ("String"=w375:string)  [unwired: 9 in, 1 out]
                n214 = Unbundle(w374) -> (w370:string[])
                n215 = Match First String(2:w370, 3:w375) -> (0:w371:i32)  [unwired: 1 out]
                n216 = property on="Test Ring" class="Ring (strict)"("Value"=w371, "Strings []"=w370) -> ()  [unwired: 2 in, 2 out]
                n217 = property on="Test Ring" class="Ring (strict)"("Visible"=TRUE) -> ()  [unwired: 2 in, 2 out]
                n218 = property on="Test Slider" class="Slide (strict)"("Visible"=FALSE) -> ()  [unwired: 2 in, 2 out]
              }
              frame "Exposure Priority  **" {
                n219 = Index Array(array=w382, index=3) -> (element=w383:cluster{string[]})
                n220 = call <vilib>:"NT Read String.vi"("Name"=w385) -> ("String"=w384:string)  [unwired: 9 in, 1 out]
                n221 = Unbundle(w383) -> (w379:string[])
                n222 = Match First String(2:w379, 3:w384) -> (0:w380:i32)  [unwired: 1 out]
                n223 = property on="Test Ring" class="Ring (strict)"("Value"=w380, "Strings []"=w379) -> ()  [unwired: 2 in, 2 out]
                n224 = property on="Test Ring" class="Ring (strict)"("Visible"=TRUE) -> ()  [unwired: 2 in, 2 out]
                n225 = property on="Test Slider" class="Slide (strict)"("Visible"=FALSE) -> ()  [unwired: 2 in, 2 out]
              }
              frame "Color Enable  **" {
                n226 = Index Array(array=w391, index=4) -> (element=w392:cluster{string[]})
                n227 = call <vilib>:"NT Read String.vi"("Name"=w394) -> ("String"=w393:string)  [unwired: 9 in, 1 out]
                n228 = Unbundle(w392) -> (w388:string[])
                n229 = Match First String(2:w388, 3:w393) -> (0:w389:i32)  [unwired: 1 out]
                n230 = property on="Test Ring" class="Ring (strict)"("Value"=w389, "Strings []"=w388) -> ()  [unwired: 2 in, 2 out]
                n231 = property on="Test Ring" class="Ring (strict)"("Visible"=TRUE) -> ()  [unwired: 2 in, 2 out]
                n232 = property on="Test Slider" class="Slide (strict)"("Visible"=FALSE) -> ()  [unwired: 2 in, 2 out]
              }
              frame Default {
                n233 = property on="Test Ring" class="Ring (strict)"("Visible"=FALSE) -> ()  [unwired: 2 in, 2 out]
                n234 = property on="Test Slider" class="Slide (strict)"("Visible"=FALSE) -> ()  [unwired: 2 in, 2 out]
              }
              frame "Brightness  **", "Color Level  **", "Compression  **", "FPS  **", "Sharpness  **" {
                n235 = call <vilib>:"NT Read Number.vi"("Name"=w400) -> ("Numeric"=w399:dbl)  [unwired: 9 in, 1 out]
                n236 = local write "Test Slider"(w399) -> ()
                n237 = property on="Test Slider" class="Slide (strict)"("Visible"=TRUE, "Scale.Maximum"=100.0 ("Scale.Range:Maximum")) -> ()  [unwired: 2 in, 2 out]
                n238 = property on="Test Ring" class="Ring (strict)"("Visible"=FALSE) -> ()  [unwired: 2 in, 2 out]
              }
            }
          }
        }
        n239 = property on="Progress" class="Clust (strict)"("Visible"=FALSE) -> ()  [unwired: 2 in, 2 out]
      }
      event "Test Name": Mouse Enter {
        # "Populate the ring with the list of tests"
        n240 = event-data() -> ()  [unwired: 1 in, 1 out]
        n241 = call <vilib>:"NT Read String Array.vi"("Name"="/TestMode/TestList") -> ("String Array"=w408:string[])  [unwired: 9 in, 1 out]
        n242 = Build Array (concatenate)("Select the test to run...", w408) -> (w407:string[])
        n243 = property on="Test Name" class="Ring (strict)"("Strings []"=w407) -> ()  [unwired: 2 in, 2 out]
      }
      event "Test Name": Value Change {
        w410 = FALSE ("Visible")
        # "Tell the robot the test name to run"
        n244 = event-data() -> ("NewVal"=w414:u16)  [unwired: 1 in]
        n245 = property on="Test Name" class="Ring (strict)"() -> ("Strings []"=w415:string[])  [unwired: 2 in, 2 out]
        n246 = local write "Progress"(T6 {"Test Progress"=0, "Test Progress Text"=""} ("Progress")) -> ()
        n247 = Index Array(array=w415, index=w414) -> (element=w413:string)
        n248 = call <vilib>:"NT Write String.vi"("String"=w413, "Name"="/TestMode/TestName") -> ()  [unwired: 9 in, 1 out]
        n249 = property on="Progress" class="Clust (strict)"("Visible"=TRUE) -> ()  [unwired: 2 in, 2 out]
        n250 = property on="Motor" class="Clust (strict)"("Visible"=w410) -> ()  [unwired: 2 in, 2 out]
        n251 = property on="Test Slider" class="Slide (strict)"("Visible"=w410) -> ()  [unwired: 2 in, 2 out]
        n252 = property on="On/Off" class="Bool (strict)"("Visible"=w410) -> ()  [unwired: 2 in, 2 out]
        n253 = property on="Rev/Fwd" class="Clust (strict)"("Visible"=w410) -> ()  [unwired: 2 in, 2 out]
        n254 = property on="Test Ring" class="Ring (strict)"("Visible"=w410) -> ()  [unwired: 2 in, 2 out]
      }
      event "Select Auto": Mouse Enter {
        # "Populate the combo box with the list of autonomous options"
        n255 = event-data() -> ()  [unwired: 1 in, 1 out]
        n256 = call <vilib>:"NT Read String Array.vi"("Name"="Auto List") -> ("String Array"=w417:string[])  [unwired: 9 in, 1 out]
        n257 = property on="Select Auto" class="CmbBox"("Strings[]"=w417) -> ()  [unwired: 2 in, 2 out]
      }
      event "Select Auto": Value Change {
        # "User modified the Auto Selection. Write to NT variable so robot knows."
        n258 = event-data() -> ("NewVal"=w420:string)  [unwired: 1 in]
        n259 = call <vilib>:"NT Write String.vi"("String"=w420, "Name"="Auto Selector") -> ()  [unwired: 9 in, 1 out]
      }
      event "Command Selection": Value Change {
        # "Get the params and show in table"
        n260 = event-data() -> ("NewVal"=w426:i32)  [unwired: 1 in]
        n261 = property on="Command Selection" class="MCListbox (strict)"() -> ("ItemNames"=w424:string[][])  [unwired: 2 in, 2 out]
        n262 = call <vilib>:"WPI_DashboardUpdate Command Params.vi"("NewVal"=w426, "Commands"=w424, "Param Tbl"=w425) -> ()  [unwired: 8 in, 1 out]
      }
      event "Execute Command": Value Change {
        # "Started one, Unique ID holds\nresponse"
        n263 = event-data() -> ()  [unwired: 1 in, 1 out]
        n264 = property on="Command Selection" class="MCListbox (strict)"() -> ("ItemNames"=w437:string[][])  [unwired: 2 in, 2 out]
        n265 = Index Array(array=w437, index (row)="Command Selection", index (col)=0) -> (element=w435:string)
        n266 = call <vilib>:"Invoke Commands.vi"("Command Params"="Command Params", "Function Name"=w435) -> ("Params"=w431:u8, "Started"=w430:bool)  [unwired: 7 in, 1 out]
        n267 = Array Subset(array="Command Params", length (row)=w431) -> (w432:string[][])  [unwired: 3 in]
        n268 = Select(t="Executing" ("Cmd Status"), s=w430, f="" ("Cmd Status")) -> (s? t:f=→"Cmd Status":string)
      }
      event "Command Selection": Double Click {
        n269 = event-data() -> ("Row"=w445:i32)  [unwired: 1 in]
        n270 = property on="Command Selection" class="MCListbox (strict)"() -> ("ItemNames"=w448:string[][])  [unwired: 2 in, 2 out]
        n271 = local read "Command Params"() -> (w444:string[][])
        n272 = Index Array(array=w448, index (row)=w445, index (col)=0) -> (element=w446:string)
        n273 = call <vilib>:"Invoke Commands.vi"("Command Params"=w444, "Function Name"=w446) -> ("Params"=w443:u8, "Started"=w438:bool)  [unwired: 7 in, 1 out]
        n274 = Array Subset(array=w444, length (row)=w443) -> (w442:string[][])  [unwired: 3 in]
        n275 = Select(t="Executing" ("Cmd Status"), s=w438, f="" ("Cmd Status")) -> (s? t:f=w439:string)
        n276 = local write "Cmd Status"(w439) -> ()
      }
      event "CheckList": Double Click {
        # "Shift clears all"
        # "Update symbols on the listbox"
        n277 = event-data() -> ("PlatMods.Shift"=w450:bool, "Row"=w452:i32)  [unwired: 1 in]
        n278 = case shown="True" w450 {
          tunnel: w452 -> [w456 _]
          tunnel: 1 -> [w455 _]
          frame False {
            n279 = property on="CheckList" class="LstBox (strict)"() -> ("Item Symbols"=w454:i32[])  [unwired: 2 in, 2 out]
            n280 = Replace Array Subset(array=w454, new element=w455, index=w456) -> (w453:i32[])
            n281 = property on="CheckList" class="LstBox (strict)"("Item Symbols"=w453) -> ()  [unwired: 2 in, 2 out]
          }
          frame True {
            w457 = 0 ("Top Row")
            n282 = property on="CheckList" class="LstBox (strict)"() -> ("Number of Rows"=w459:u32)  [unwired: 2 in, 2 out]
            n283 = Initialize Array(0, w459) -> (w458:i32[])
            n284 = property on="CheckList" class="LstBox (strict)"("Top Row"=w457, "Value"=w457, "Item Symbols"=w458) -> ()  [unwired: 2 in, 2 out]
          }
        }
      }
      event "CheckList": Key Down {
        # "Update symbols on the listbox\nLeft and right keys check and uncheck"
        n285 = event-data() -> ("VKey"=w463:T25)  [unwired: 1 in]
        n286 = case shown="\"Left\", \"Right\"" w463 {
          selector: w463 -> [w468 _]
          tunnel: eventvkey."Left" ("VKey") -> [w466 _]
          frame "Left", "Right" {
            n287 = Equal?(x=w466, y=w468) -> (x = y?=w467:bool)
            n288 = Select(t=0, s=w467, f=1) -> (s? t:f=w469:i32)
            n289 = property on="CheckList" class="LstBox (strict)"() -> ("Item Symbols"=w472:i32[])  [unwired: 2 in, 2 out]
            n290 = Replace Array Subset(array=w472, new element=w469, index="CheckList") -> (w471:i32[])
            n291 = property on="CheckList" class="LstBox (strict)"("Item Symbols"=w471) -> ()  [unwired: 2 in, 2 out]
          }
          frame Default {
          }
        }
      }
      event "Motor.Enable": Value Change {
        # "When the test mode otor enable helper is set, update that\ntree row item's value"
        n292 = event-data() -> ("NewVal"=w478:bool)  [unwired: 1 in]
        n293 = Unbundle("Motor") -> ("Value"=w477:dbl)  [unwired: 1 out]
        n294 = Select(t=w477, s=w478, f=0.0) -> (s? t:f=w475:dbl)
        n295 = call <vilib>:"NT Write Number.vi"("Numeric"=w475, "Name"=w474) -> ()  [unwired: 9 in, 1 out]
      }
      event "Test Slider": Value Change {
        # "When the test mode slider helper is set, update that\ntree row item's value"
        n296 = event-data() -> ("NewVal"=w481:dbl)  [unwired: 1 in]
        n297 = call <vilib>:"NT Write Number.vi"("Numeric"=w481, "Name"=w482) -> ()  [unwired: 9 in, 1 out]
      }
      event "On/Off": Value Change {
        # "When the test mode on/off helper value is set, update that\ntree row item's value"
        n298 = event-data() -> ("NewVal"=w486:bool)  [unwired: 1 in]
        n299 = Boolean To (0,1)(Boolean=w486) -> (0, 1=w485:i16)
        n300 = call <vilib>:"NT Write Number.vi"("Numeric"=w485, "Name"=w484) -> ()  [unwired: 9 in, 1 out]
      }
      event "Rev/Fwd": Value Change {
        # "When the test mode helper value for relays is set, update that\ntree row item's value"
        n301 = event-data() -> ("NewVal.Forward"=w494:bool, "NewVal.Reverse"=w493:bool)  [unwired: 1 in]
        n302 = Boolean To (0,1)(Boolean=w494) -> (0, 1=w490:i16)
        n303 = Boolean To (0,1)(Boolean=w493) -> (0, 1=w492:i16)
        n304 = Negate(x=w492) -> (-x=w491:i16)
        n305 = Add(x=w490, y=w491) -> (x+y=w489:i16)
        n306 = call <vilib>:"NT Write Number.vi"("Numeric"=w489, "Name"=w488) -> ()  [unwired: 9 in, 1 out]
      }
      event "Test Ring": Value Change {
        # "When a test mode helper value is selected from the ring,\nset the tree item's variable to the string value"
        n307 = event-data() -> ("NewVal"=w498:u16)  [unwired: 1 in]
        n308 = property on="Test Ring" class="Ring (strict)"() -> ("Strings []"=w499:string[])  [unwired: 2 in, 2 out]
        n309 = Index Array(array=w499, index=w498) -> (element=w497:string)
        n310 = call <vilib>:"NT Write String.vi"("String"=w497, "Name"=w496) -> ()  [unwired: 9 in, 1 out]
      }
      event "Rec Mode": Value Change {
        # "Update globals for recording mode and path to read log from.\nClear when logging and let NetworkTables set path for vision to\nuse."
        n311 = event-data() -> ("NewVal"=w510:enum32{"Stop", "Record", "Playback"})  [unwired: 1 in]
        n312 = global write "WPI_DashboardLogging Global.vi" "Logging Filename"(path "") -> ()
        n313 = global write "WPI_DashboardLogging Global.vi" "Recording"(w510) -> ()
        n314 = case shown="\"Playback\"" w510 {
          tunnel: w509 -> [_ w512 w521]
          tunnel: [_ _ w520] -> w507
          tunnel: [_ _ w519] -> _
          tunnel: w505 -> [_ _ w517]
          tunnel: cluster{i32, i32} {-250, 170} -> [_ _ w516]
          tunnel: [_ _ T26 {"Image Size"=TRUE, "Image Type"=TRUE, "Pixel Value"=TRUE, "ROI Information"=TRUE, "Zoom Factor"=FALSE} ("Image Information Shown:All Elements")] -> w503
          tunnel: [_ _ TRUE ("Zoom Factor")] -> w502
          tunnel: w501 -> [_ _ w513]
          frame Default {
          }
          frame "Stop", "Record" {
            # "Place Window too"
            n315 = invoke class="VI" method="FP.Close"(reference=w512) -> (reference out=w511:refnum<vi>)  [unwired: 2 in, 2 out]
            n316 = invoke class="VI" method="Abort VI"(reference=w511) -> ()  [unwired: 2 in, 3 out]
          }
          frame "Playback" {
            n317 = call "Open Playback Panel.vi"("Offset"=w516, "DB VI Ref"=w517, "Playback in"=w521) -> ("Playback out"=w518:refnum<vi>)  [unwired: 8 in]
            n318 = register-events(w518, w513) -> (reference out=w520:refnum<event-registration>, error out=w519:errorcluster)  [unwired: 2 in]
          }
        }
        n319 = property on="Camera Image" class="ImageControl"("Image Information Shown"=w503, "Image Information Visible"=w502) -> ()  [unwired: 2 in, 2 out]
        n320 = call <vilib>:"WPI_DashboardNT Log FieldName Cache.vi"("Operation"=enum16{"Lookup/Add", "Index", "Clear"}."Clear") -> ()  [unwired: 8 in, 3 out]
      }
      event Panel Close {
        w523 = enum32{"Stop", "Record", "Playback"}."Stop" ("Rec Mode")
        # "Playback window has been closed, abort"
        n321 = event-data() -> ()  [unwired: 1 in, 4 out]
        n322 = local write "Rec Mode"(w523) -> ()
        n323 = global write "WPI_DashboardLogging Global.vi" "Recording"(w523) -> ()
      }
      event Panel Close {
        # "Abort playback window and ourself"
        n324 = event-data() -> ()  [unwired: 1 in, 4 out]
        n325 = invoke class="VI" method="FP.Close"(reference=w527) -> (reference out=w526:refnum<vi>)  [unwired: 2 in, 2 out]
        n326 = invoke class="VI" method="Abort VI"(reference=w526) -> (error out=w525:errorcluster)  [unwired: 2 in, 2 out]
        n327 = invoke class="VI" method="Abort VI"(error in=w525) -> ()  [unwired: 2 in, 3 out]
      }
      event User Event {
        n328 = event-data() -> ("IDs"=w534:cluster{"RPC field ID":u16, "Unique ID":u16}, "String"=w533:string)  [unwired: 1 in]
        n329 = Bundle("IDs"=w534, "String"=w533) -> (w532:T8)  [unwired: 1 in]
        n330 = call <vilib>:"Retrieve RPC Response.vi"("RPC Response"=w532) -> ("Output"=w530:string[][])  [unwired: 10 in]
        n331 = Build Array (concatenate)(w528, w530) -> (w529:string[][])
        n332 = local write "Command Params"(w529) -> ()
        n333 = local write "Cmd Status"("" ("Cmd Status")) -> ()
      }
      event "Tree": Double Click {
        n334 = event-data() -> ("PlatMods"=w538:T29, "Tag"=w537:string)  [unwired: 1 in]
        n335 = Unbundle(w538) -> ("Shift"=w536:bool)  [unwired: 4 out]
        n336 = Not(x=w536) -> (.not. x?=w535:bool)
        n337 = call <vilib>:"NT Update Persistence.vi"("Persistence"=w535, "Name"=w537) -> ()  [unwired: 9 in, 1 out]
      }
    }
  }
  n338 = while {
    tunnel: w61 -> [w541]
    i -> [w544]
    stop <- FALSE stop-if-true
    n339 = Wait (ms)(milliseconds to wait=u32 100) -> ()  [unwired: 1 out]
    n340 = case shown="\"Playback\"" "Rec Mode" {
      tunnel: w544 -> [_ _ w559]
      tunnel: [u32 2829099 ("Base Color") u32 11141120 ("Target Color") w548] -> w540
      frame "Stop", Default {
        # "Reset the color, extra updates don't cost much"
      }
      frame "Record" {
      }
      frame "Playback" {
        # "Playback"
        n341 = Quotient & Remainder(x=w559, y=u32 50 ("milliseconds to wait")) -> (x-y*floor(x/y)=w555:u32)  [unwired: 1 out]
        n342 = Divide(x=w555, y=u32 50 ("milliseconds to wait")) -> (x/y=w552:dbl)
        n343 = Multiply(x=6.283185307179586, y=w552) -> (x*y=w557:dbl)
        n344 = Sine(x=w557) -> (sin(x)=w556:dbl)
        n345 = Absolute Value(x=w556) -> (abs(x)=w549:dbl)
        n346 = call "Interpolate RGB Color.vi"("Proportion"=w549, "Target Color"=u32 30976, "Base Color"=u32 2829099) -> ("Result Color"=w548:u32)  [unwired: 8 in]
      }
    }
    n347 = property class="Pane"(reference=w541, "PaneColor"=w540) -> ()  [unwired: 1 in, 2 out]
  }
  n348 = local write "Dashboard Tab"(T2."Drive" ("Dashboard Tab")) -> ()
  n349 = property on="On/Off" class="Bool (strict)"("Visible"=w30) -> ()  [unwired: 2 in, 2 out]
  n350 = property on="Motor" class="Clust (strict)"("Visible"=w30) -> ()  [unwired: 2 in, 2 out]
  n351 = property on="Progress" class="Clust (strict)"("Visible"=w30) -> ()  [unwired: 2 in, 2 out]
  n352 = property on="Test Ring" class="Ring (strict)"("Visible"=w30) -> ()  [unwired: 2 in, 2 out]
  n353 = property on="Rev/Fwd" class="Clust (strict)"("Visible"=w30) -> ()  [unwired: 2 in, 2 out]
  n354 = while {
    tunnel: u16 1741 ("timeout ms (25000)") -> [w561]
    stop <- FALSE stop-if-true
    n355 = TCP Create Listener(10:w561) -> (0:w560:errorcluster, 3:w562:refnum<k5>)  [unwired: 4 in, 1 out]
    n356 = case shown="No Error" w560 {
      selector: w560 -> [w564 _]
      tunnel: w562 -> [w565 _]
      frame No Error {
        n357 = while {
          tunnel: w565 -> [w568]
          tunnel: w564 -> [w567]
          stop <- FALSE stop-if-true
          n358 = TCP Wait On Listener(8:w567, 11:w568) -> (0:w569:errorcluster, 4:w570:refnum<k5>)  [unwired: 2 in, 3 out]
          n359 = local write "TCP"(w570) -> ()
          n360 = case shown="No Error" w569 {
            frame No Error {
            }
            frame Error {
              n361 = Wait (ms)(milliseconds to wait=u32 1000) -> ()  [unwired: 1 out]
            }
          }
        }
      }
      frame Error {
        n362 = Wait (ms)(milliseconds to wait=u32 1000) -> ()  [unwired: 1 out]
      }
    }
  }
  n363 = local write "Command Selection"(u16 0 ("milliseconds to wait")) -> ()
  n364 = local write "Command Params"(string[][] [] ("Command Params")) -> ()
  n365 = global write "WPI_DashboardLogging Global.vi" "Recording"(w55) -> ()
  n366 = local write "Rec Mode"(w55) -> ()
  n367 = disable-structure shown="Disabled" {
    frame Disabled {
      n368 = case shown="\"Boiler\"" {
        selector: _ -> [_]
        tunnel: _ -> [w580]
        tunnel: [w576] -> _
        tunnel: _ -> [w575]
        tunnel: [w573] -> _
        tunnel: [w574] -> _
        frame "Boiler" {
          w578 = 70.0  # Score Cutoff
          w582 = 5.0  # Particles
          w581 = 0.04  # Size Limit %
          # "Boiler code"
          # "HSV threshold"
          n369 = call "Boiler2"("Image In"=w575) -> ("Image Out"=w573:T5, "error out"=w583:errorcluster)  [unwired: 25 in]
          n370 = call <vilib>:"Clear Errors.vi"("error in (no error)"=w583) -> ()  [unwired: 5 in, 2 out]
          n371 = call "Sorted Particle Report 2016.vi"("Min Area Size %"=w581, "Particle Count Limit"=w582, "Pixel Measurements"=w580, "Image in"=w573) -> ("Sorted Data"=w579:dbl[][])  [unwired: 1 out]
          n372 = call "Cull and Group Boiler.vi"("Score Cutoff"=w578, "Sorted Data"=w579) -> ("Rect"=w574:T22, "Center"=w577:cluster{"X":dbl, "Y":dbl})  [unwired: 6 in, 2 out]
          n373 = Unbundle By Name(w577) -> ("X"=w576:dbl)
        }
      }
    }
    frame Enabled {
    }
  }
  n374 = call <vilib>:"NT Write String.vi"("String"="Select Auto", "Name"="Auto Selector") -> ()  [unwired: 9 in, 1 out]
